vi "Read FIFO.vi"(8 "error in (no error)":errorcluster, 9 "timeout in ms (0)":i32 format="%d ms", 11 "Pool in":refnum<class "Pool.lvclass">) -> (0 "error out":errorcluster, 1 "timed out?":bool, 2 "element":i32, 3 "Pool out":refnum<class "Pool.lvclass">)   [LabVIEW 2017, in "DSF Core.lvlib" / "Pool.lvclass"]
uses:
  Pool.lvclass
  Pool.lvclass/Pool.ctl
  Debug/FIFO Flags/FIFO Flags.lvclass/FIFO Flags.ctl
  Debug/FIFO Flags/FIFO Flags.lvclass
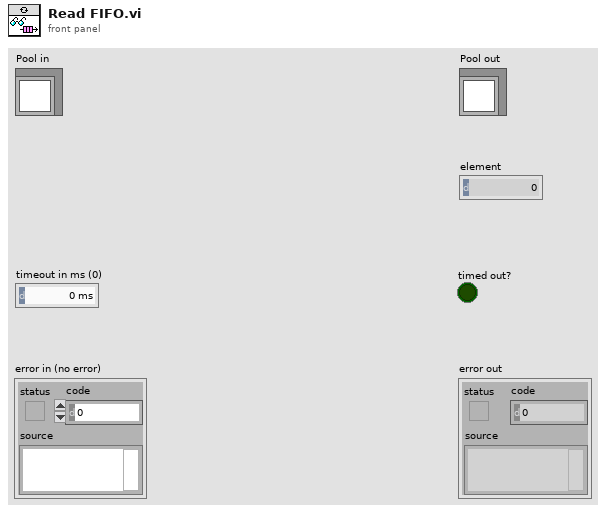
[diagram p1: front panel]
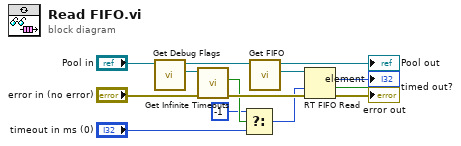
[diagram p0: block diagram]
diagram:
  n1 = call "Get Debug Flags.vi"("Pool in"="Pool in") -> ("FIFO Debug Flags"=w7:refnum<class "FIFO Flags.lvclass">, "Pool out"=w3:refnum<class "Pool.lvclass">)  [unwired: 9 in]
  n2 = call "Get Infinite Timeouts.vi"("FIFO Debug Flags in"=w7) -> ("infinite timeouts"=w6:bool)  [unwired: 9 in, 1 out]
  n3 = Select(t=-1, s=w6, f="timeout in ms (0)") -> (s? t:f=w2:i32)
  n4 = call "Get FIFO.vi"("Pool in"=w3) -> ("FIFO"=w12:refnum<k33>, "Pool out"=→"Pool out":refnum<class "Pool.lvclass">)  [unwired: 9 in]
  n5 = RT FIFO Read(0:w12, 2:w2, 3:"error in (no error)") -> (9:→"element":i32, 10:→"timed out?":bool, 11:→"error out":errorcluster)  [unwired: 1 in, 2 out]
